vi "testSelectState(s)NoError_Error.vi"(8 "error in (no error)":errorcluster, 11 "testStateMachineUtilities in":refnum<class "testStateMachineUtilities.lvclass">) -> (0 "error out":errorcluster, 3 "testStateMachineUtilities out":refnum<class "testStateMachineUtilities.lvclass">)   [LabVIEW 2013, in "testStateMachineUtilities.lvclass"]
uses:
  testStateMachineUtilities.lvclass
  source/State Machine Support API/Select State(s)_err.vi
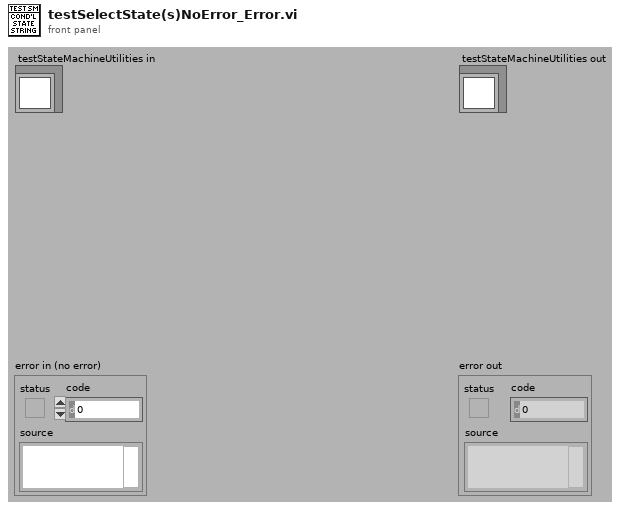
[diagram p1: front panel]
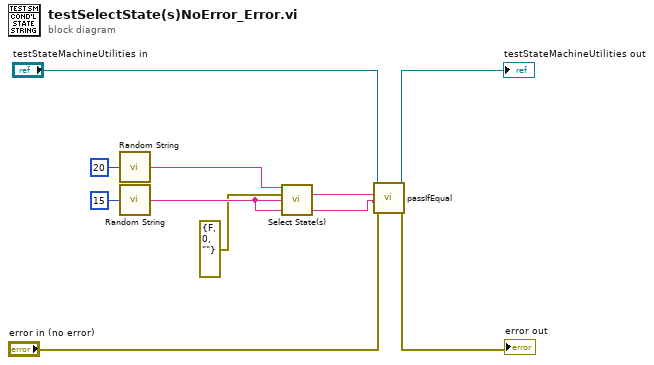
[diagram p0: block diagram]
diagram:
  n1 = call "Random String.vi"("Length"=20) -> ("ASCII"=w3:string)  [unwired: 4 in]
  n2 = call "Random String.vi"("Length"=15) -> ("ASCII"=w2:string)  [unwired: 4 in]
  n3 = call-poly "Select State(s).vi"("State(s) if True (\"\")"=w3, "Select"=errorcluster {"status"=FALSE, "code"=0, "source"=""}, "State(s) if False (\"\")"=w2) -> ("States Out"=w4:string)  [unwired: 12 in]
  n4 = call-dynamic "passIfEqual.vi"("error in (no error)"="error in (no error)", "y"=w2, "x"=w4, "TestCase in"="testStateMachineUtilities in") -> ("error out"=→"error out":errorcluster, "TestCase out"=→"testStateMachineUtilities out":refnum<class "testStateMachineUtilities.lvclass">)  [unwired: 6 in]
